vi "Define 1D Wave PDE IC (Numeric).vi"(0 "PDE in":refnum<class "NI_PDE.lvclass">, 5 "Initial Condition":dbl[](array[numeric]), 7 "type":T1 items=["Value", "Derivative"], 11 "error in (no error)":errorcluster) -> (4 "PDE out":refnum<class "NI_PDE.lvclass">, 15 "error out":errorcluster)   [LabVIEW 2017, in "NI_PDE.lvlib"]
doc: "Defines the initial condition of a partial differential equation. You must manually select the polymorphic instance to use."
uses:
  <vilib>/gmath/NI_PDE.lvlib
  <vilib>/gmath/pde.llb/Common/PDE_IC Type.ctl
  <vilib>/gmath/pde.llb/PDEClass/NI_PDE.lvclass
  <vilib>/gmath/pde.llb/ICClass/IC_1D_Numeric/NI_IC_1D_Numeric.lvclass
  e:/builds/penguin/labview/branches/2017/dev/dist/vi.lib/gmath/pde.llb/ICClass/NI_IC.lvclass
  <vilib>/gmath/pde.llb/PDEClass/PDE_Wave_1D/NI_PDE_Wave_1D.lvclass
  e:/builds/penguin/labview/branches/2017/dev/dist/vi.lib/gmath/pde.llb/PDEClass/NI_PDE.lvclass
  <vilib>/gmath/pde.llb/ICClass/IC_1D_Numeric/IC Data.ctl
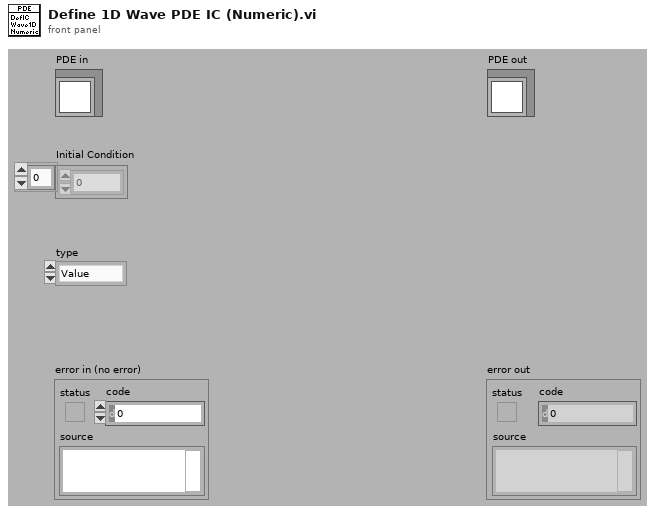
[diagram p1: front panel]
types:
  T1 = typedef "NI_PDE.lvlib/PDE_IC Type.ctl" = i32
  T2 = typedef "NI_PDE.lvlib/NI_IC_1D_Numeric.lvclass/IC Data.ctl" = cluster{"type":T1, "H":dbl[]}
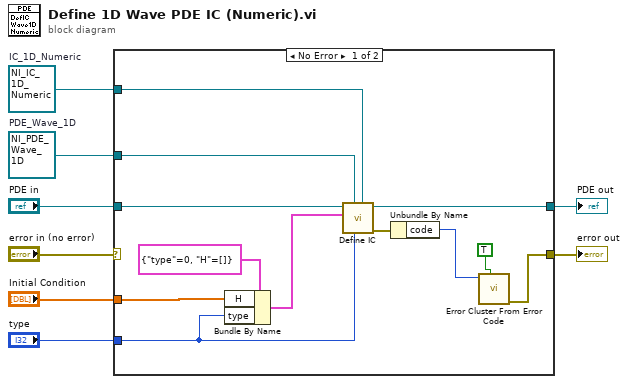
[diagram p0: block diagram]
diagram:
  w2 = refnum<class "NI_PDE_Wave_1D.lvclass"> refnum  # PDE_Wave_1D
  w1 = refnum<class "NI_IC_1D_Numeric.lvclass"> refnum  # IC_1D_Numeric
  n1 = case shown="No Error" "error in (no error)" {
    selector: "error in (no error)" -> [_ w22]
    tunnel: "PDE in" -> [w17 w21]
    tunnel: [w16 w21] -> w7
    tunnel: "type" -> [w12 _]
    tunnel: "Initial Condition" -> [w13 _]
    tunnel: [w18 w22] -> w4
    tunnel: w2 -> [w10 _]
    tunnel: w1 -> [w9 _]
    frame No Error {
      n2 = Bundle By Name(cluster=T2 {"type"=0, "H"=[]} ("IC data"), "H"=w13, "type"=w12) -> (w11:T2)
      n3 = call <vilib>:"Define IC.vi"("target IC"=w9, "index"=w12, "target PDE"=w10, "IC"=w11, "PDE in"=w17) -> ("error out"=w15:errorcluster, "PDE out"=w16:refnum<class "NI_PDE.lvclass">)  [unwired: 2 in, 3 out]
      n4 = Unbundle By Name(w15) -> ("code"=w20:i32)
      n5 = call <vilib>:"Error Cluster From Error Code.vi"("show call chain? (False)"=TRUE, "error code (0)"=w20) -> ("error out"=w18:errorcluster)  [unwired: 1 in, 6 out]
    }
    frame Error {
    }
  }
  "PDE out" <- w7
  "error out" <- w4
